vi "FTW-VIServer-OSinfo.vi"(11 "error in":errorcluster) -> (4 "OS Display Name":string, 6 "OS Name":string, 8 "OS Version":string, 15 "error out":errorcluster)   [LabVIEW 2015]
panel:
  # "Inputs"
  # "Outputs"
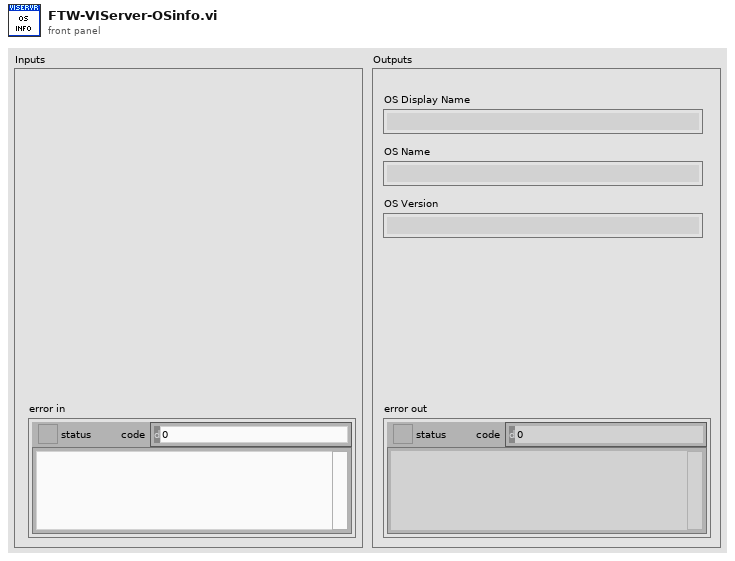
[diagram p1: front panel]
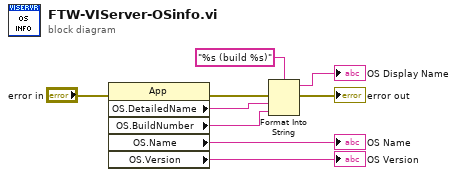
[diagram p0: block diagram]
diagram:
  n1 = property class="App"(error in="error in") -> (error out=w5:errorcluster, "OS.DetailedName"=w2:string, "OS.BuildNumber"=w1:string, "OS.Name"=→"OS Name":string, "OS.Version"=→"OS Version":string)  [unwired: 1 in, 1 out]
  n2 = Format Into String(format string="%s (build %s)", error in=w5, w2, w1) -> (resulting string=→"OS Display Name":string, error out=→"error out":errorcluster)  [unwired: 1 in]
